vi "encoder safety.vi"(0 "Desired Rate":dbl, 1 "Forward Limit":dbl, 2 "Reverse Limit":dbl, 3 "Cutoff Rate":dbl=0.2, 5 "Min Rate":dbl, 6 "Encoder Refnum":string) -> (7 "Encoder Disconnected":bool, 9 "No Rate Read":bool, 11 "At Distance Limit":bool, 13 "Encoder Directional Issue":bool, 14 "Rate Output":dbl, 19 "Input Out of Range":bool)   [LabVIEW 2014]
doc: "This VI provides two types of safety for your motors. An encoder for the motor is required. If the encoder reference is innalid, the motor won't be allowed to run. \nThe first safetyis a distance limit. The forward and reverse limit parameters specify the max and min valus for the encoder distance to read until the motor is stopped and only allowed to move away from its limit. \nThe second safety is an encoder safety. The Cutoff Rate parameter is the maximum value allowed to be sent to the motor without a response seen from the encoder. So, if the code is trying to set a value higher than this parameter and the encoder doesn't register a response, the motor will be disabled. It will be reenabled when movement is registered from the encoder. This safety will also permanately disable the motor if the encoder reads some inanely high rate. Consider a replacement...."
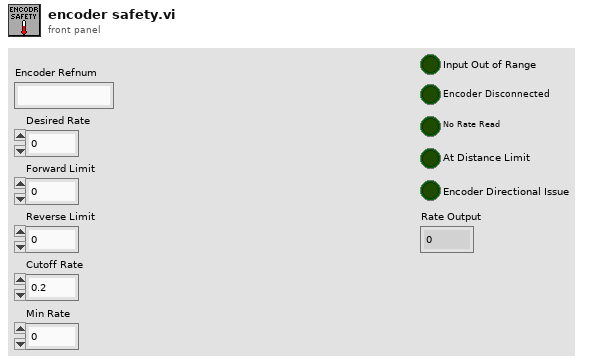
[diagram p1: front panel]
types:
  T1 = typedef "WPI_EncoderDevRef.ctl" = cluster{"DevStatus":errorcluster, "EncoderIndex":T2, "CounterIndex":T3, "DistancePerCount":dbl, "Decoding Type":T4}
  T2 = typedef "FPGA_EncoderIdx.ctl" = enum8{"Enc 0", "Enc 1", "Enc 2", "Enc 3", "Enc 4", "Enc 5", "Enc 6", "Enc 7", "Invalid"}
  T3 = typedef "FPGA_CounterCtrSystemIndex.ctl" = enum8{"Ctr 0", "Ctr 1", "Ctr 2", "Ctr 3", "Ctr 4", "Ctr 5", "Ctr 6", "Ctr 7", "Invalid"}
  T4 = typedef "WPI_EncoderType.ctl" = enum16{"1x", "2x", "4x"}
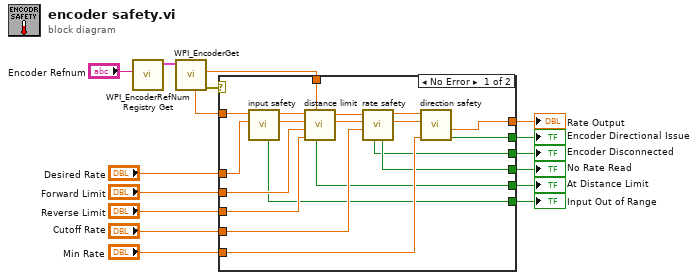
[diagram p0: block diagram]
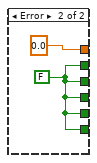
[diagram p2: hidden frame]
diagram:
  n1 = call <vilib>:"WPI_EncoderRefNum Registry Get.vi"("refnum name"="Encoder Refnum") -> ("EncoderDevRef"=w15:T1)  [unwired: 9 in, 1 out]
  n2 = call <vilib>:"WPI_EncoderGet.vi"("EncoderDevRef"=w15) -> ("error out"=w7:errorcluster, "Distance"=w12:dbl, "Rate"=w14:dbl)  [unwired: 5 in, 3 out]
  n3 = case shown="No Error" w7 {
    tunnel: w14 -> [w25 _]
    tunnel: "Desired Rate" -> [w21 _]
    tunnel: w12 -> [w33 _]
    tunnel: [w30 0.0 ("Output Rate")] -> w11
    tunnel: "Forward Limit" -> [w22 _]
    tunnel: "Reverse Limit" -> [w23 _]
    tunnel: "Cutoff Rate" -> [w29 _]
    tunnel: [w18 w36] -> w6
    tunnel: [w19 w36] -> w5
    tunnel: "Min Rate" -> [w27 _]
    tunnel: [w35 w36] -> w3
    tunnel: [w20 w36] -> w2
    tunnel: [w17 w36] -> w1
    frame No Error {
      n4 = call "input safety.vi"("Desired Rate"=w21, "Encoder Rate"=w25) -> ("Safe Rate"=w24:dbl, "Encoder Rate Out"=w26:dbl, "Input Out of Range"=w17:bool)  [unwired: 7 in]
      n5 = call "distance limit.vi"("Encoder Rate"=w26, "Encoder Distance"=w33, "Desired Rate"=w24, "Forward Limit"=w22, "Reverse Limit"=w23) -> ("At Distance Limit"=w20:bool, "Encoder Rate Out"=w34:dbl, "Output Rate"=w28:dbl)  [unwired: 1 in]
      n6 = call "rate safety.vi"("Cutoff Rate"=w29, "Desired Rate"=w28, "Encoder Rate"=w34) -> ("Output Rate"=w31:dbl, "Encoder Rate Out"=w32:dbl, "No Rate Read"=w19:bool, "Encoder Failure"=w18:bool)  [unwired: 5 in]
      n7 = call "direction safety.vi"("Min Rate"=w27, "Desired Rate"=w31, "Encoder Rate"=w32) -> ("Encoder Directional Issue"=w35:bool, "Super Safe Rate"=w30:dbl)  [unwired: 2 in, 1 out]
    }
    frame Error {
      w36 = FALSE ("Cutoff Tripped")
    }
  }
  "Rate Output" <- w11
  "Encoder Disconnected" <- w6
  "No Rate Read" <- w5
  "Encoder Directional Issue" <- w3
  "At Distance Limit" <- w2
  "Input Out of Range" <- w1
